vi "Main.vi"() -> ()   [LabVIEW 2010]
uses:
  <vilib>/MDSplus/Classes/Tree_Class/Tree.lvclass
  <vilib>/MDSplus/Classes/Data_Class/TreeNode_Class/TreeNode.lvclass
  <vilib>/MDSplus/Library/MDSplus.lvlib
panel:
  out "error out":errorcluster
  out "message":string=" INSTRUCTIONS:\r\rNormal Use:  When using subVIs that incorporate the error in/error out (or error I/O) structure, place this handler where you want to inform the user of an error, typically at the end of the I/O data path, as the last action of the program.  If the error in error? is ERROR, the handler creates a message describing the error and its source.  If the type of dialog = 1 (default), the message is displayed to the user, who can only acknowedge it.  If the type = 2, the user can acknowledge the message or abort execution; aborting a program with active I/O is not recommended.  If the type = 0, no message is displayed; this is used to process the error programmatically, and the error out cluster elements are wired to individual terminals for that reason.  \r\rOther Use:\n\r\nlocal testing.  To test the error code of a subVI or function that does not have the error I/O structure, you can wire its error code and a source string to the local error code and error source inputs.  If error in error? indicates no error and error code is not equal to 0, the local code and source are substituted for the error in values, and error? is set TRUE (ERROR)."
  out "source out":string
  out "Size out":i64
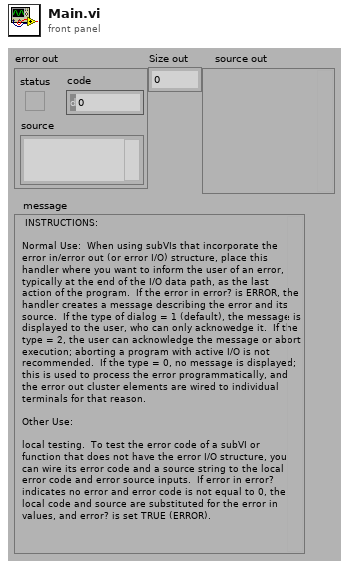
[diagram p1: front panel]
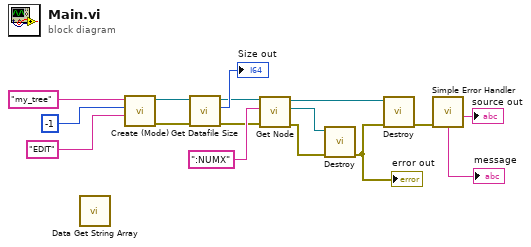
[diagram p0: block diagram]
diagram:
  n1 = call <vilib>:"Data Get String Array.vi"() -> ()  [unwired: 8 in, 4 out]
  n2 = call <vilib>:"Create (Mode).vi"("Mode"="EDIT", "Shot"=-1, "Name"="my_tree") -> ("error out"=w3:errorcluster, "Tree out"=w14:refnum<class "Tree.lvclass">)  [unwired: 7 in]
  n3 = call-dynamic "Get Datafile Size.vi"("error in (no error)"=w3, "Tree in"=w14) -> ("error out"=w2:errorcluster, "Size out"=→"Size out":i64, "Tree out"=w11:refnum<class "Tree.lvclass">)  [unwired: 7 in]
  n4 = call-dynamic "Get Node.vi"("error in (no error)"=w2, "Path"=":NUMX", "Tree in"=w11) -> ("error out"=w1:errorcluster, "Node out"=w7:refnum<class "TreeNode.lvclass">, "Tree out"=w9:refnum<class "Tree.lvclass">)  [unwired: 6 in]
  n5 = call-dynamic "Destroy.vi"("error in (no error)"=w1, "TreeNode in"=w7) -> ("error out"=w6:errorcluster)  [unwired: 9 in]
  "error out" <- w6
  n6 = call-dynamic "Destroy.vi"("error in (no error)"=w6, "Tree in"=w9) -> ("error out"=w8:errorcluster)  [unwired: 9 in]
  n7 = call <vilib>:"Simple Error Handler.vi"("error in (no error)"=w8) -> ("source out"=→"source out":string, "message"=→"message":string)  [unwired: 4 in, 3 out]
